vi "Attach Role Policy.vi"(8 "error in (no error)":errorcluster, 9 "Policy ARN":string, 10 "Role Name":string, 11 "IAM Session in":refnum<class "IAM Session.lvclass">) -> (0 "error out":errorcluster, 3 "IAM Session out":refnum<class "IAM Session.lvclass">)   [LabVIEW 2015, in "NI_AWS_IAM.lvlib" / "IAM Session.lvclass"]
uses:
  IAM Session.lvclass
  Core/HTTP Request/Response.ctl
  Core/HTTP Request/Request Options.ctl
  Core/HTTP Request/Name Value Pair.ctl
  Core/HTTP Request/Region handling.ctl
  Core/HTTP Request/URL formatting.ctl
  Core/HTTP Request/HTTP Request.lvclass
panel:
  out "Response":T1
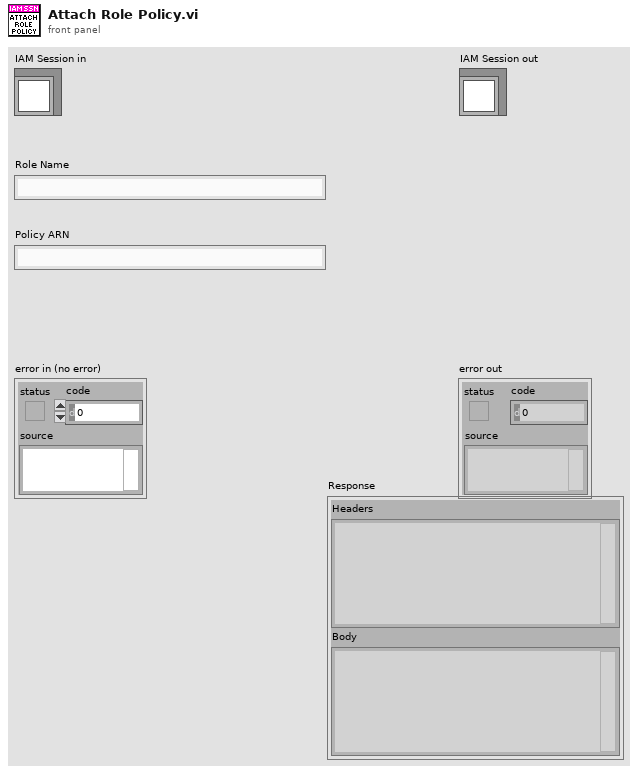
[diagram p1: front panel]
types:
  T1 = typedef "NI_AWS_Core.lvlib/HTTP Request.lvclass/Response.ctl" = cluster{"Headers":string, "Body":string}
  T2 = typedef "NI_AWS_Core.lvlib/HTTP Request.lvclass/Name Value Pair.ctl" = cluster{"name":string, "value":string}
  T3 = typedef "NI_AWS_Core.lvlib/HTTP Request.lvclass/Request Options.ctl" = cluster{"request headers":T2[], "request parameters":T2[], "request body":string, "region handling":T4, "URL formatting":T5}
  T4 = typedef "NI_AWS_Core.lvlib/HTTP Request.lvclass/Region handling.ctl" = enum16{"use region everywhere", "use region (authentication only)", "use region (URL only)", "ignore region everwhere"}
  T5 = typedef "NI_AWS_Core.lvlib/HTTP Request.lvclass/URL formatting.ctl" = enum16{"region-", "region."}
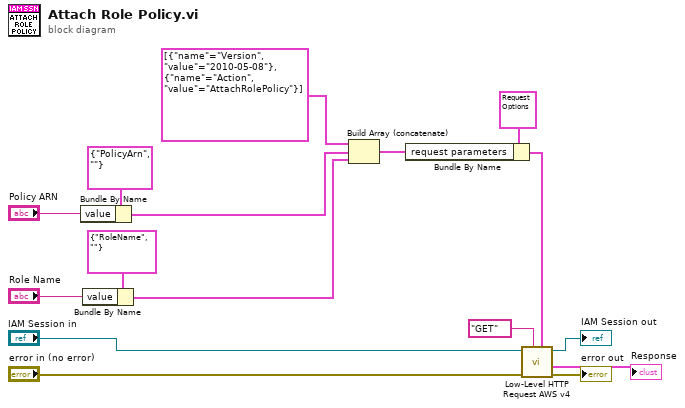
[diagram p0: block diagram]
diagram:
  n1 = Bundle By Name(cluster=T2 {"name"="PolicyArn", "value"=""} ("Name Value Pair"), "value"="Policy ARN") -> (w3:T2)
  n2 = Bundle By Name(cluster=T2 {"name"="RoleName", "value"=""} ("Name Value Pair"), "value"="Role Name") -> (w2:T2)
  n3 = Build Array (concatenate)(T2[] [{"name"="Version", "value"="2010-05-08"}, {"name"="Action", "value"="AttachRolePolicy"}], w3, w2) -> (w8:T2[])
  n4 = Bundle By Name(cluster=T3 {"request headers"=[], "request parameters"=[], "request body"="", "region handling"=enum."use region everywhere", "URL formatting"=enum."region."} ("Request Options"), "request parameters"=w8) -> (w10:T3)
  n5 = call "Low-Level HTTP Request AWS v4.vi"("Request Options"=w10, "HTTP-Verb"="GET", "error in (no error)"="error in (no error)", "AWS Core in"="IAM Session in") -> ("error out"=→"error out":errorcluster, "Response"=→"Response":T1, "AWS Core out"=→"IAM Session out":refnum<class "IAM Session.lvclass">)  [unwired: 4 in, 1 out]
